vi "DP I-O Init Level (F1L1).vi"(0 "StimGen":T1, 1 "DP Freqs":T2, 5 "DP stimulus params":T3={"Start (dB)"=20.0, "Stop (dB)"=80.0, "Step (dB)"=10.0, "Ear"=enum."Left", "f2 (kHz)"="", "f1"=0.0, "f1 mode"=enum."re f2", "L1"=0.0, "L1 mode"=enum."re L2"}, 11 "error in (no error)":errorcluster) -> (3 "StimGen Out":T1, 4 "Multipliers (2D)":dbl[][](array[numeric]), 6 "Gains (2D)":dbl[][](array[numeric]), 14 "Nominal f2 SPL":dbl[](array[numeric]), 15 "error out":errorcluster)   [LabVIEW 2020]
uses:
  Typedefs/DP-Stim Params (F1L1).ctl
  epl-vi-lib/Utility VIs/Type Defs/Left-Right ring.ctl
  Typedefs/DP-StimGen.ctl
  Typedefs/DP-Freqs.ctl
  epl-vi-lib/Utility VIs/Math VIs/LinSpace (start-stop-step).vi
  epl-vi-lib/PXI DAQ VIs/DAQ Engine VIs/AO Gain and Multiplier VIs/PXI Multipliers to AO Gains (1D).vi
  epl-cal-vi-lib/CIE-2 Tone.vi
panel:
  out "Max SPL 2":dbl
  out "Max SPL 1":dbl
  out "Nominal f1 SPL":dbl[](array[numeric])
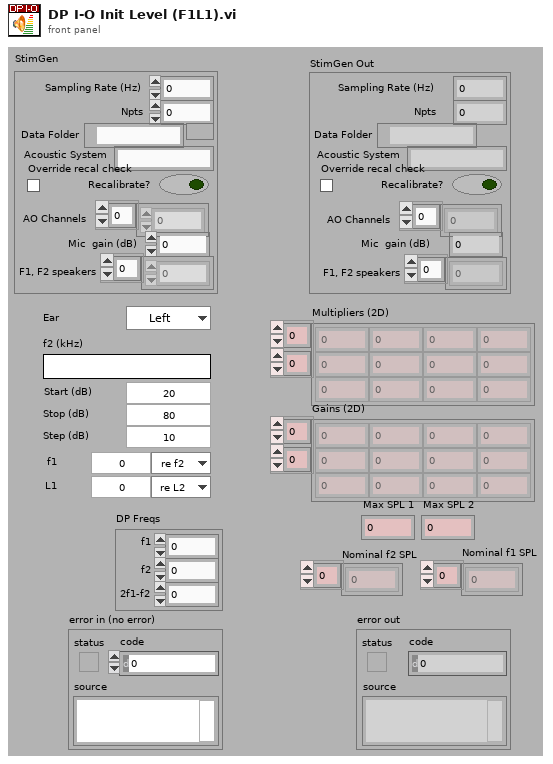
[diagram p1: front panel]
types:
  T1 = typedef "DP-StimGen.ctl" = cluster{"Sampling Rate (Hz)":dbl, "Npts":i32, "Data Folder":path, "Acoustic System":string, "Recalibrate?":bool, "AO Channels":i32[], "Mic  gain (dB)":dbl, "F1, F2 speakers":i32[], "Override recal check":bool}
  T2 = typedef "DP-Freqs.ctl" = cluster{"f1":dbl, "f2":dbl, "2f1-f2":dbl}
  T3 = typedef "DP-Stim Params (F1L1).ctl" = cluster{"Start (dB)":dbl, "Stop (dB)":dbl, "Step (dB)":dbl, "Ear":T4, "f2 (kHz)":string, "f1":dbl, "f1 mode":enum16{"re f2", "kHz"}, "L1":dbl, "L1 mode":enum16{"re L2", "dB"}}
  T4 = typedef "Left-Right ring.ctl" = enum16{"Right", "Left"}
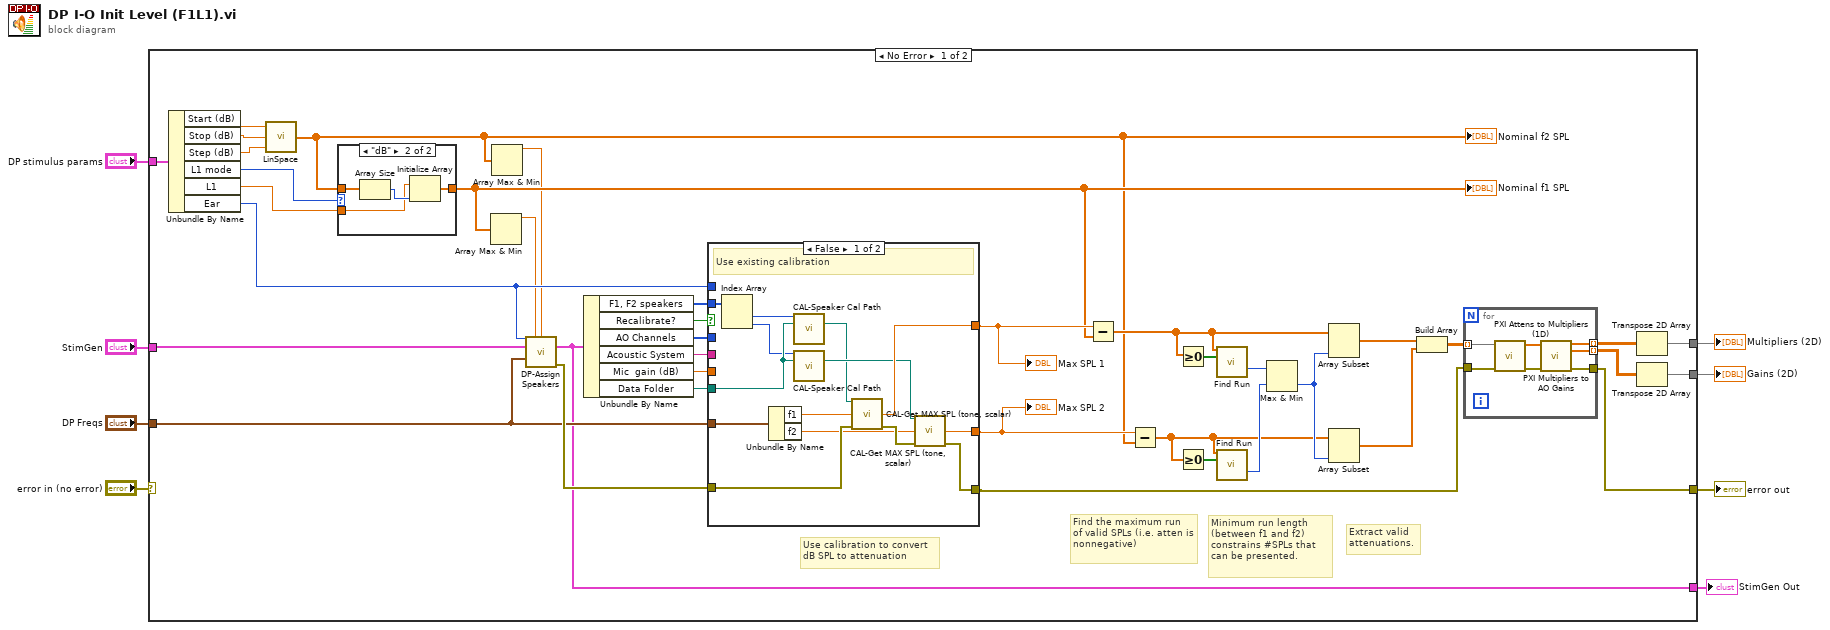
[diagram p0: block diagram]
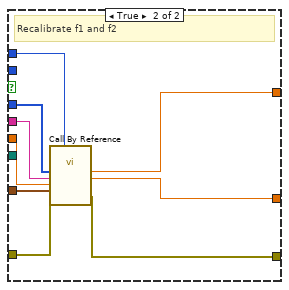
[diagram p2: hidden frame]
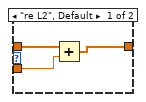
[diagram p3: hidden frame]
diagram:
  n1 = case shown="No Error" "error in (no error)" {
    selector: "error in (no error)" -> [_ w85]
    tunnel: "DP stimulus params" -> [w15 _]
    tunnel: [w40 w85] -> w7
    tunnel: [w35 _] -> w5
    tunnel: [w34 _] -> w4
    tunnel: "DP Freqs" -> [w17 _]
    tunnel: "StimGen" -> [w16 _]
    tunnel: [w14 _] -> w1
    frame No Error {
      # "Use calibration to convert\ndB SPL to attenuation"
      # "Extract valid attenuations."
      # "Minimum run length (between f1 and f2) constrains #SPLs that can be presented."
      # "Find the maximum run\nof valid SPLs (i.e. atten is nonnegative)"
      n2 = Unbundle By Name(w15) -> ("Start (dB)"=w47:dbl, "Stop (dB)"=w46:dbl, "Step (dB)"=w45:dbl, "L1 mode"=w28:enum16{"re L2", "dB"}, "L1"=w29:dbl, "Ear"=w11:T4)
      n3 = call-poly "LinSpace.vi"("Step"=w45, "Stop"=w46, "Start"=w47) -> ("Array"=w12:dbl[])  [unwired: 1 in, 1 out]
      "Nominal f2 SPL" <- w12
      n4 = case shown="\"dB\"" w28 {
        tunnel: w12 -> [w73 w77]
        tunnel: [w72 w76] -> w13
        tunnel: w29 -> [w71 w74]
        frame "re L2", Default {
          n5 = Add(x=w73, y=w71) -> (x+y=w72:dbl[])
        }
        frame "dB" {
          n6 = Array Size(array=w77) -> (size(s)=w75:i32)
          n7 = Initialize Array(w74, w75) -> (w76:dbl[])
        }
      }
      "Nominal f1 SPL" <- w13
      n8 = Array Max & Min(array=w13) -> (max value=w10:dbl)  [unwired: 3 out]
      n9 = Array Max & Min(array=w12) -> (max value=w9:dbl)  [unwired: 3 out]
      n10 = call "DP-Assign Speakers.vi"("Ear"=w11, "F1 Max Req"=w10, "F2 Max  Req"=w9, "StimGen In"=w16, "DP Freqs"=w17) -> ("StimGen Out"=w14:T1, "error out"=w23:errorcluster)  [unwired: 7 in, 2 out]
      n11 = Unbundle By Name(w14) -> ("F1, F2 speakers"=w22:i32[], "Recalibrate?"=w27:bool, "AO Channels"=w21:i32[], "Acoustic System"=w25:string, "Mic  gain (dB)"=w24:dbl, "Data Folder"=w26:path)
      n12 = case shown="False" w27 {
        tunnel: w23 -> [w61 w70]
        tunnel: [w59 w68] -> w18
        tunnel: [w58 w69] -> w20
        tunnel: w26 -> [w57 _]
        tunnel: w11 -> [_ w66]
        tunnel: [w54 w67] -> w19
        tunnel: w25 -> [_ w63]
        tunnel: w24 -> [_ w64]
        tunnel: w22 -> [w51 _]
        tunnel: w17 -> [w48 w65]
        tunnel: w21 -> [_ w62]
        frame False {
          # "Use existing calibration"
          n13 = Index Array(array=w51) -> (element #1=w53:i32, element #2=w52:i32)  [unwired: 2 in]
          n14 = Unbundle By Name(w48) -> ("f1"=w50:dbl, "f2"=w49:dbl)
          n15 = call "CAL-Speaker Cal Path.vi"("Speaker"=w53, "Data Folder"=w57) -> ("Cal Path"=w55:path)  [unwired: 12 in, 1 out]
          n16 = call "CAL-Speaker Cal Path.vi"("Speaker"=w52, "Data Folder"=w57) -> ("Cal Path"=w56:path)  [unwired: 12 in, 1 out]
          n17 = call "CAL-Get MAX SPL (tone, scalar).vi"("Cal Path"=w55, "Frequency (kHz)"=w50, "error in (no error)"=w61) -> ("Max SPL"=w58:dbl, "error out"=w60:errorcluster)  [unwired: 11 in]
          n18 = call "CAL-Get MAX SPL (tone, scalar).vi"("Cal Path"=w56, "Frequency (kHz)"=w49, "error in (no error)"=w60) -> ("Max SPL"=w54:dbl, "error out"=w59:errorcluster)  [unwired: 11 in]
        }
        frame True {
          # "Recalibrate f1 and f2"
          n19 = call-by-ref "?"("AO Channels"=w62, "Ear"=w66, "Acoustic System"=w63, "Probe mic gain (dB)"=w64, "DP Freqs"=w65, "error in (no error)"=w70) -> ("Max SPL1"=w69:dbl, "Max SPL2"=w67:dbl, "error out"=w68:errorcluster)  [unwired: 9 in, 2 out]
        }
      }
      "Max SPL 1" <- w20
      "Max SPL 2" <- w19
      n20 = Subtract(x=w20, y=w13) -> (x-y=w33:dbl[])
      n21 = Subtract(x=w19, y=w12) -> (x-y=w32:dbl[])
      n22 = Greater Or Equal To 0?(x=w33) -> (x >= 0?=w44:bool[])
      n23 = Greater Or Equal To 0?(x=w32) -> (x >= 0?=w30:bool[])
      n24 = call "Find Run.vi"("Array"=w33, "Condition"=w44) -> ("Run length"=w43:i32)  [unwired: 10 in, 3 out]
      n25 = call "Find Run.vi"("Array"=w32, "Condition"=w30) -> ("Run length"=w42:i32)  [unwired: 10 in, 3 out]
      n26 = Max & Min(x=w43, y=w42) -> (min(x,y)=w41:i32)  [unwired: 1 out]
      n27 = Array Subset(array=w33, length=w41) -> (w37:dbl[])  [unwired: 1 in]
      n28 = Array Subset(array=w32, length=w41) -> (w31:dbl[])  [unwired: 1 in]
      n29 = Build Array(w37, w31) -> (w36:dbl[][])
      n30 = for {
        tunnel: w18 -> [w84]
        tunnel: [w83] -> w40
        tunnel: [w82] -> w39 mode=indexing
        tunnel: [w81] -> w38 mode=indexing
        tunnel: w36 -> [w78] mode=indexing
        n31 = call "PXI Attens to Multipliers (1D).vi"("error in (no error)"=w84, "Array of Attens"=w78) -> ("error out"=w79:errorcluster, "Multiplier setting"=w80:dbl[])  [unwired: 8 in]
        n32 = call-poly "PXI Multipliers to AO Gains.vi"("Multipliers in"=w80, "error in (no error)"=w79) -> ("Multipliers out"=w82:dbl[], "Gains"=w81:dbl[], "error out"=w83:errorcluster)  [unwired: 11 in]
      }
      n33 = Transpose 2D Array(2D array=w39) -> (transposed array=w35:dbl[][])
      n34 = Transpose 2D Array(2D array=w38) -> (transposed array=w34:dbl[][])
    }
    frame Error {
    }
  }
  "error out" <- w7
  "Multipliers (2D)" <- w5
  "Gains (2D)" <- w4
  "StimGen Out" <- w1
